vi "Solve2.vi"(8 "Error In":errorcluster, 11 "object in":refnum<class "2024_12.lvclass">) -> (0 "Error Out":errorcluster, 2 "Result":u64, 3 "object out":refnum<class "2024_12.lvclass">)   [LabVIEW 2023, in "2024_12.lvclass"]
uses:
  2024_12.lvclass
  2024_12.lvclass/2024_12.ctl
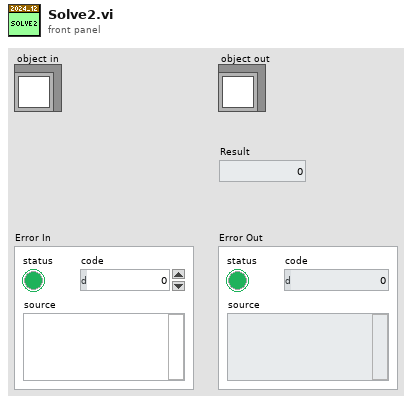
[diagram p1: front panel]
types:
  T1 = cluster{u8, cluster{i32, i32}, "PixelsFound":cluster{"x":i32, "y":i32}[]}[]
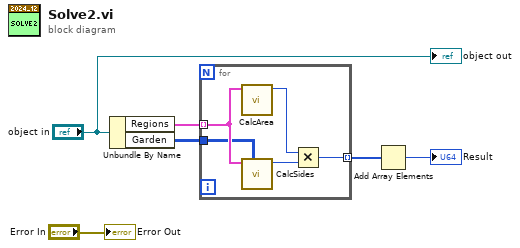
[diagram p0: block diagram]
diagram:
  n1 = Unbundle By Name("object in") -> ("Regions"=w2:T1, "Garden"=w1:u8[][])
  n2 = for {
    tunnel: w2 -> [w11] mode=indexing
    tunnel: [w9] -> w5 mode=indexing
    tunnel: w1 -> [w8]
    n3 = call "CalcArea.vi"("Cluster"=w11) -> ("Numeric"=w7:u64)  [unwired: 10 in]
    n4 = call "CalcSides.vi"("Garden"=w8, "Cluster"=w11) -> ("Numeric"=w10:u64)  [unwired: 9 in]
    n5 = Multiply(x=w7, y=w10) -> (x*y=w9:u64)
  }
  n6 = Add Array Elements(numeric array=w5) -> (sum=→"Result":u64)
  "Error Out" <- "Error In"
  "object out" <- "object in"
